vi "Destruct.vi"(8 "Error in (no error)":errorcluster, 11 "LogWriterMock in":refnum<class "LogWriterMock.lvclass">) -> (0 "Error out":errorcluster, 2 "Array log out":T1[](array[typedef]) {"Priority" items=["EMERGENCY", "ALERT", "CRITICAL", "ERROR", "WARNING", "NOTICE", "INFO", "DEBUG"]})   [LabVIEW 2011, in "LogWriterMock.lvclass"]
uses:
  LogWriterMock.lvclass
  Log/LogCluster.ctl
  Log/PrioritiesRing.ctl
  Log/Log.lvclass
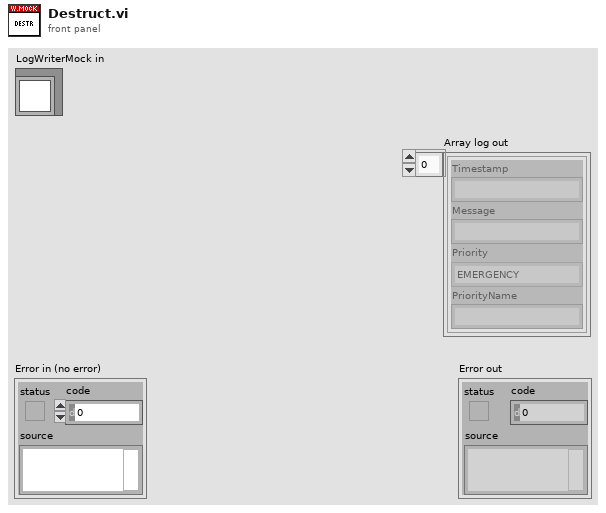
[diagram p1: front panel]
types:
  T1 = typedef "Log.lvclass/LogCluster.ctl" = cluster{"Timestamp":string, "Message":string, "Priority":T2, "PriorityName":string}
  T2 = typedef "Log.lvclass/PrioritiesRing.ctl" = u32
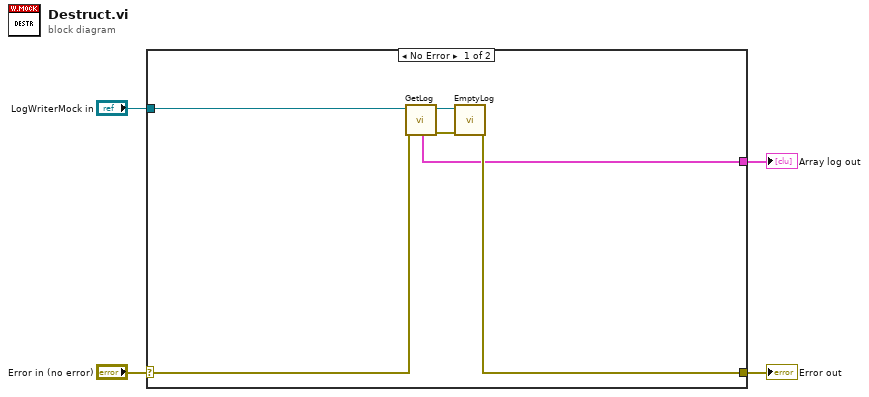
[diagram p0: block diagram]
diagram:
  n1 = case shown="No Error" "Error in (no error)" {
    selector: "Error in (no error)" -> [w8 w11]
    tunnel: [w7 w11] -> w3
    tunnel: "LogWriterMock in" -> [w9 _]
    tunnel: [w5 _] -> w1
    frame No Error {
      n2 = call "GetLog.vi"("Error in (no error)"=w8, "LogWriterMock in"=w9) -> ("Error out"=w6:errorcluster, "Array log out"=w5:T1[], "LogWriterMock out"=w10:refnum<class "LogWriterMock.lvclass">)  [unwired: 7 in]
      n3 = call "EmptyLog.vi"("Error in (no error)"=w6, "LogWriterMock in"=w10) -> ("Error out"=w7:errorcluster)  [unwired: 8 in, 1 out]
    }
    frame Error {
    }
  }
  "Error out" <- w3
  "Array log out" <- w1
